vi "Random_Array.vi"() -> ()   [LabVIEW 2022 SP3]
uses:
  <vilib>/numeric/sub_Random U32.vi
  <vilib>/numeric/Random Number (Range) I64.vi
panel:
  in  "N":dbl
  out "Random 0-N":dbl[](array[numeric])
  # "Random_Array:\nEnter a value of N to create an array of length N+1,\ncontaining values 0-N in a random order."
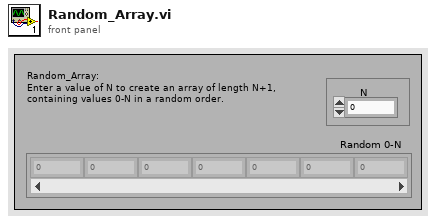
[diagram p1: front panel]
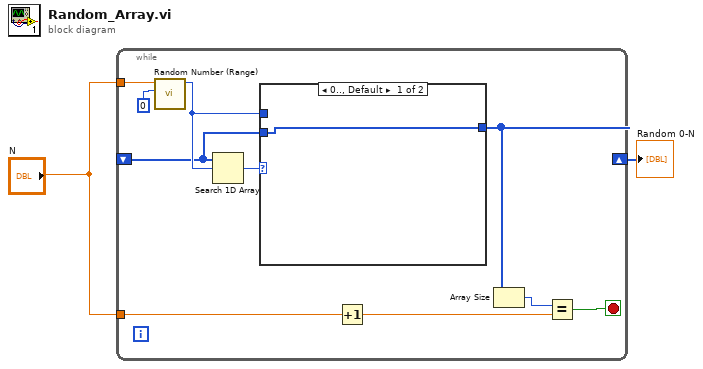
[diagram p0: block diagram]
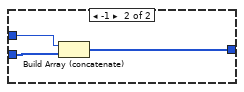
[diagram p2: hidden frame]
diagram:
  n1 = while {
    shift-right: [w8] -> w2
    shift-left: _ -> [w10]
    tunnel: "N" -> [w9]
    tunnel: "N" -> [w6]
    stop <- w4 stop-if-true
    n2 = call-poly <vilib>:"Random Number (Range).vi"("lower bound (-100)"=0, "upper bound (100)"=w9) -> ("number"=w11:i64)  [unwired: 9 in]
    n3 = Search 1D Array(1D array=w10, element=w11) -> (index of element=w12:i32)  [unwired: 1 in]
    n4 = case shown="0.., Default" w12 {
      tunnel: w11 -> [_ w16]
      tunnel: w10 -> [w13 w15]
      tunnel: [w13 w14] -> w8
      frame 0.., Default {
      }
      frame -1 {
        n5 = Build Array (concatenate)(w16, w15) -> (w14:i64[])
      }
    }
    n6 = Increment(x=w6) -> (x+1=w5:dbl)
    n7 = Array Size(array=w8) -> (size(s)=w7:i32)
    n8 = Equal?(x=w7, y=w5) -> (x = y?=w4:bool)
  }
  "Random 0-N" <- w2
